vi "SVFA Zoom Cross Spectrum (Real-Im).vi"(0 "scaled signal X [EUx]":waveform(dbl)={"t0"=timestamp(0 s since 1904-01-01), "dt"=1e-05, "Y"=[]}, 1 "scaled signal Y [EUy]":waveform(dbl)={"t0"=timestamp(0 s since 1904-01-01), "dt"=1e-05, "Y"=[]}, 3 "zoom settings":T7={"frequency range"={"start frequency"=1000.0, "stop frequency"=2000.0}, "window"=1, "number of lines"=400, "% overlap"=0.0} {"% overlap" min=0.0 format="%.2f"; "number of lines" min=2; "window" items=["None ", "Hanning", "Hamming", "Blackman-Harris", "Exact Blackman", "Blackman", "Flat Top", "4 Term B-Harris ", "7 Term B-Harris", "Low Sidelobe"]; "frequency range"."stop frequency" min=0.0 format="%.2f"; "frequency range"."start frequency" min=0.0 format="%.2f"}, 5 "error in (no error)":errorcluster, 7 "averaging parameters":T9={"averaging mode"=enum."No averaging", "weighting mode"=enum."Exponential", "number of averages"=10, "linear mode"=enum."One shot"} {"number of averages" min=1 step=1}, 9 "restart averaging (F)":bool) -> (11 "averaging done":bool, 12 "new spectrum available":bool, 13 "averages completed":dbl, 14 "real part [EUx EUy rms]":cluster{"f0":dbl, "df":dbl, "real part":dbl[]} {"real part" format="%.2p"; "df" format="%.2p"; "f0" format="%.2p"}, 16 "imaginary part [EUx EUy rms]":T8 {"imaginary part" format="%.2p"; "df" format="%.2p"; "f0" format="%.2p"}, 17 "unit label":string, 18 "spectrum info":T1={"channel name"="", "description"="", "x-axis units"=1, "spectral info"={"spectrum type"=enum."Power [Magnitude^2]", "linear/dB"=enum."linear", "window"=0, "window size"=0, "FFT size"=0}, "engineering units"=0, "custom label"="", "dB reference [EU]"=0.0, "peak units"=enum."rms", "weighting filter"=0, "spectral density?"=FALSE, "unit label"="", "spectrum skewed?"=FALSE, "complimentary spectrum units"=enum."none"} {"x-axis units" items=["Time (s)"=0, "Frequency-CB (Hz)"=1, "Frequency-CPB (Hz)"=1248, "Frequency-Arbitrary (Hz)"=2357, "Quefrency (s)"=2, "Revolutions (rev)"=3, "Order"=4, "Speed (RPM)"=11, "Speed (rad/s)"=21, "Index"=65535]; "weighting filter" items=["Linear", "A-weighting", "B-weighting", "C-weighting", "ITU-R 468-4", "Dolby", "CCITT", "C-message", "Wb", "Wc", "Wd", "We", "Wf", "Wh", "Wj", "Wk", "Wm", "AES17 20 kHz lowpass", "AES17 40 kHz lowpass", "AES17 20 kHz highpass", "AES17 40 kHz highpass"]; "dB reference [EU]" format="%.2f"; "engineering units" items=["custom..."=0, "V"=1, "A"=21, "C"=30, "pC"=31, "s"=32, "-"=29, "Pa"=2, "N"=20, "g"=3, "m/s^2"=4, "m/s"=5, "m"=6, "mm/s"=12, "mm"=13, "micron/s"=14, "micron"=15, "in/s^2"=7, "in/s"=8, "in"=9, "mil/s"=10, "mil"=11, "rad/s^2"=16, "rad/s"=17, "rad"=18, "deg/s^2"=26, "deg/s"=27, "deg"=28, "RPM"=22, "cycle/s^2"=23, "Hz"=24, "cycle"=25, "strain"=19]; "spectral info"."window" items=["None "=0, "Hanning"=1, "Hamming"=2, "Blackman-Harris"=3, "Exact Blackman"=4, "Blackman"=5, "Flat Top"=6, "4 Term B-Harris "=7, "7 Term B-Harris"=8, "Low Sidelobe"=9, "Force - Exponential"=10, "Gaussian"=62]}, 19 "error out":errorcluster)   [LabVIEW 2017]
doc: "Computes the zoom cross power spectrum of <B>scaled signal X [EUx]</B>, <B>scaled signal Y [EUy]</B>, and <B>zoom settings</B>. Results are returned as real part and imaginary part. Data accumulates each time the VI is called. However, it returns a new spectrum only when sufficient data accumulates. Indicators and subsequent processing should only be called when <B>new spectrum available</B> is TRUE."
uses:
  <vilib>/addons/_NISVFA/_Shared subVIs/Controls/svc_Spectrum Info.ctl
  <vilib>/addons/_NISVFA/_Shared subVIs/Controls/svc_X-Axis Units.ctl
  <vilib>/addons/_NISVFA/_Shared subVIs/Controls/svc_Spectrum Type.ctl
  <vilib>/addons/_NISVFA/_Shared subVIs/Controls/svc_Engineering Units Text Ring.ctl
  <vilib>/addons/_NISVFA/_Shared subVIs/Controls/svc_Weighting Filter Text Ring.ctl
  <vilib>/addons/_NISVFA/_Shared subVIs/Controls/svc_Complimentary Spectrum Units.ctl
  <vilib>/addons/_NISVFA/_Shared subVIs/Spectrum Averaging/svfa_Reset Averaging State Info.vi
  <vilib>/addons/_NISVFA/_Shared subVIs/Spectrum Averaging/svfa_Average Array with Avg Checks (complex) No State.vi
  <vilib>/addons/_NISVFA/_Shared subVIs/Spectrum Averaging/svfa_Average Array (complex) No State.vi
  <vilib>/addons/_NISVFA/_Shared subVIs/Spectrum Averaging/svfa_No Average Array (complex).vi
  <vilib>/addons/_NISVFA/_Shared subVIs/Spectrum Averaging/svfa_Average Array (complex).vi
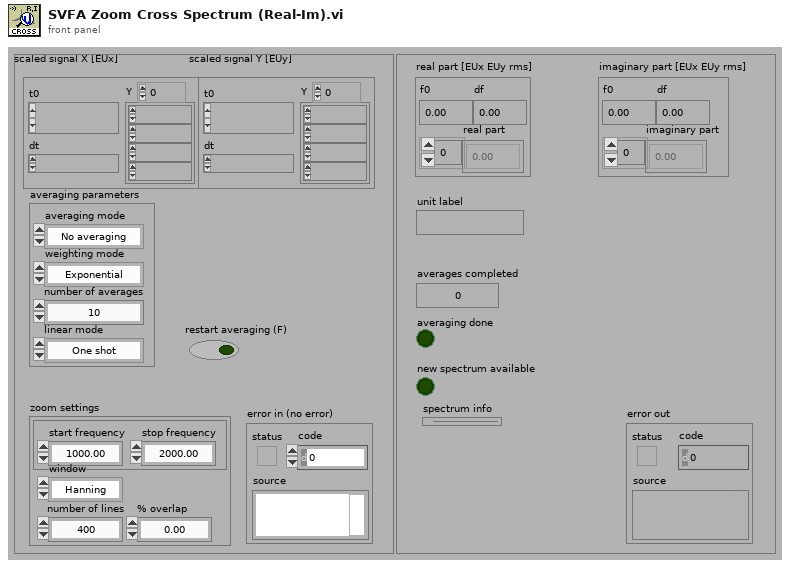
[diagram p1: front panel]
types:
  T1 = typedef "svc_Spectrum Info.ctl" = cluster{"channel name":string, "description":string, "x-axis units":T2, "spectral info":cluster{"spectrum type":T3, "linear/dB":enum16{"linear", "dB"}, "window":u16, "window size":i32, "FFT size":i32}, "engineering units":T4, "custom label":string, "dB reference [EU]":dbl, "peak units":enum16{"rms", "peak", "peak-peak"}, "weighting filter":T5, "spectral density?":bool, "unit label":string, "spectrum skewed?":bool, "complimentary spectrum units":T6}
  T2 = typedef "svc_X-Axis Units.ctl" = u16
  T3 = typedef "svc_Spectrum Type.ctl" = enum16{"FFT Spectrum [complex]", "Amplitude [Magnitude]", "Power [Magnitude^2]", "Cross Spectrum [complex]", "Frequency Response [Complex]"}
  T4 = typedef "svc_Engineering Units Text Ring.ctl" = u16
  T5 = typedef "svc_Weighting Filter Text Ring.ctl" = u16
  T6 = typedef "svc_Complimentary Spectrum Units.ctl" = enum16{"none", "radians", "degrees", "cycles", "imaginary"}
  T7 = cluster{"frequency range":cluster{"start frequency":dbl, "stop frequency":dbl}, "window":u16, "number of lines":i32, "% overlap":dbl}
  T8 = cluster{"f0":dbl, "df":dbl, "imaginary part":dbl[]}
  T9 = cluster{"averaging mode":enum16{"No averaging", "Vector averaging", "RMS averaging", "Peak hold"}, "weighting mode":enum16{"Linear", "Exponential"}, "number of averages":u32, "linear mode":enum16{"One shot", "Auto restart"}}
  T10 = enum16{"Restart processing", "Continue processing", "Skip processing"}
  T11 = enum16{"Cross spectrum", "Frequency response", "Coherent output power"}
  T12 = enum16{"No averaging", "Vector averaging", "RMS averaging", "Peak hold"}
  T13 = cluster{"zoom settings":cluster{"center frequency":dbl, "zoom":i32, "trim":dbl}, "FFT settings":cluster{"window":enum16{"None ", "Hanning", "Hamming", "Blackman-Harris", "Exact Blackman", "Blackman", "Flat Top", "4 Term B-Harris ", "7 Term B-Harris", "Low Sidelobe"}, "window size":i32, "FFT size":i32, "%overlap":dbl}}
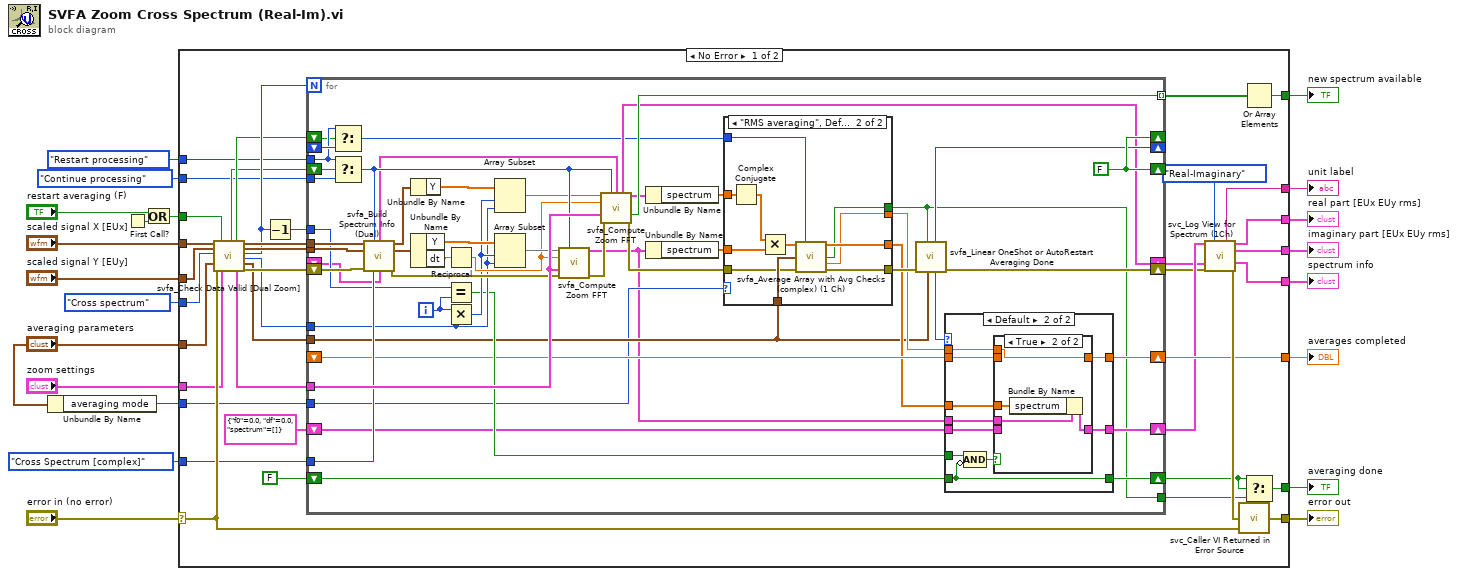
[diagram p0: block diagram]
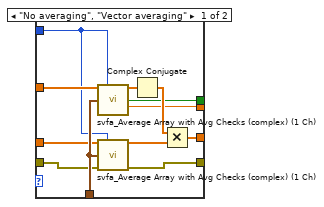
[diagram p2: hidden frame]
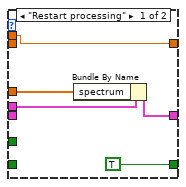
[diagram p3: hidden frame]
diagram:
  n1 = Unbundle By Name("averaging parameters") -> ("averaging mode"=w15:T12)
  n2 = First Call?() -> (First Call?: T/F=w21:bool)
  n3 = Or(x="restart averaging (F)", y=w21) -> (x .or. y?=w14:bool)
  n4 = case shown="No Error" "error in (no error)" {
    selector: "error in (no error)" -> [w50 w156]
    tunnel: "scaled signal X [EUx]" -> [w60 _]
    tunnel: "scaled signal Y [EUy]" -> [w59 _]
    tunnel: [w56 _] -> w5
    tunnel: [w55 _] -> w4
    tunnel: [w51 w156] -> w2
    tunnel: [w23 _] -> w7
    tunnel: w14 -> [w57 _]
    tunnel: "zoom settings" -> [w48 _]
    tunnel: [w25 _] -> w9
    tunnel: [w45 _] -> w8
    tunnel: [w54 _] -> w3
    tunnel: [w53 _] -> w6
    tunnel: "averaging parameters" -> [w58 _]
    tunnel: T11."Cross spectrum" ("measurement") -> [w47 _]
    tunnel: svc_Spectrum_Type."Cross Spectrum [complex]" ("spectrum type") -> [w34 _]
    tunnel: w15 -> [w33 _]
    tunnel: T10."Restart processing" ("processing control") -> [w30 _]
    tunnel: T10."Continue processing" ("processing control") -> [w29 _]
    frame No Error {
      n5 = call <vilib>:"svfa_Check Data Valid [Dual Zoom].vi"("stimulus [X]"=w60, "response [Y]"=w59, "measurement"=w47, "averaging parameters"=w58, "error in (no error)"=w50, "restart averaging (F)"=w57, "zoom settings"=w48) -> ("reset processing"=w31:bool, "restart averaging"=w32:bool, "zoom FFT settings"=w35:T13, "dup stimulus [X]"=w41:waveform(dbl), "dup response [Y]"=w40:waveform(dbl), "iterations"=w37:i32, "maximum block size"=w28:i32, "dup averaging parameters"=w38:T9, "error out"=w39:errorcluster)  [unwired: 3 in, 1 out]
      n6 = Decrement(x=w37) -> (x-1=w36:i32)
      n7 = for {
        N: w37 -> [_]
        shift-left: cluster{"f0":dbl, "df":dbl, "spectrum":cdb[]} {"f0"=0.0, "df"=0.0, "spectrum"=[]} ("FFT spectrum") -> [w77]
        shift-right: [w78] -> w44
        tunnel: w38 -> [w66]
        tunnel: [w68] -> w22
        tunnel: [w76] -> w46 mode=indexing
        tunnel: w40 -> [w106]
        tunnel: w41 -> [w107]
        shift-right: [w74] -> w43
        shift-left: _ -> [w73]
        shift-right: [w84] -> _
        shift-left: _ -> [w98]
        tunnel: w36 -> [w92]
        tunnel: w35 -> [w110]
        tunnel: w34 -> [w101]
        tunnel: w33 -> [w65]
        shift-right: [w111] -> w42
        shift-left: w39 -> [w102]
        shift-right: [w80] -> w45
        shift-left: _ -> [w79]
        shift-right: [w94] -> _
        shift-left: w32 -> [w96]
        shift-right: [w94] -> _
        shift-left: w31 -> [w100]
        tunnel: w30 -> [w97]
        tunnel: w29 -> [w99]
        tunnel: w28 -> [w85]
        shift-right: [w82] -> w24
        shift-left: FALSE ("restart averaging") -> [w81]
        i -> [w93]
        w94 = FALSE ("reset processing")
        n8 = Select(t=w97, s=w96, f=w98) -> (s? t:f=w72:T10)
        n9 = Select(t=w97, s=w100, f=w99) -> (s? t:f=w95:T10)
        n10 = call <vilib>:"svfa_Build Spectrum Info (Dual).vi"("scaled signal  X [EU]"=w107, "processing control"=w95, "scaled signal  Y [EU]"=w106, "error in (no error)"=w102, "spectrum type"=w101, "spectrum info in"=w73) -> ("spectrum info out"=w75:T1, "dup scaled signal  X [EU]"=w105:waveform(dbl), "dup scaled signal  Y [EU]"=w104:waveform(dbl), "error out"=w103:errorcluster)  [unwired: 5 in, 1 out]
        n11 = Unbundle By Name ("Get Waveform Components")(w105) -> ("Y"=w91:dbl[])
        n12 = Unbundle By Name ("Get Waveform Components")(w104) -> ("Y"=w89:dbl[], "dt"=w109:dbl)
        n13 = Reciprocal(x=w109) -> (1/x=w87:dbl)
        n14 = Equal?(x=w92, y=w93) -> (x = y?=w83:bool)
        n15 = Multiply(x=w93, y=w85) -> (x*y=w86:i32)
        n16 = Array Subset(array=w91, index=w86, length=w85) -> (w90:dbl[])
        n17 = Array Subset(array=w89, index=w86, length=w85) -> (w88:dbl[])
        n18 = call <vilib>:"svfa_Compute Zoom FFT.vi"("x"=w88, "processing control"=w95, "fs"=w87, "zoom FFT settings"=w110, "error in (no error)"=w103) -> ("FFT spectrum"=w64:cluster{"f0":dbl, "df":dbl, "spectrum":cdb[]}, "error out"=w108:errorcluster)  [unwired: 6 in, 3 out]
        n19 = call <vilib>:"svfa_Compute Zoom FFT.vi"("x"=w90, "processing control"=w95, "spectrum info"=w75, "fs"=w87, "zoom FFT settings"=w110, "error in (no error)"=w108) -> ("spectrum info out"=w74:T1, "FFT spectrum"=w62:cluster{"f0":dbl, "df":dbl, "spectrum":cdb[]}, "spectrum ready"=w76:bool, "error out"=w71:errorcluster)  [unwired: 5 in, 1 out]
        n20 = Unbundle By Name(w62) -> ("spectrum"=w61:cdb[])
        n21 = Unbundle By Name(w64) -> ("spectrum"=w63:cdb[])
        n22 = case shown="\"RMS averaging\", Default" w65 {
          tunnel: [w114 w130] -> w67
          tunnel: [w115 w131] -> w68
          tunnel: w66 -> [w118 w128]
          tunnel: w61 -> [w117 w125]
          tunnel: w63 -> [w116 w124]
          tunnel: [w122 w132] -> w69
          tunnel: w71 -> [w113 w127]
          tunnel: [w119 w126] -> w70
          tunnel: w72 -> [w112 w129]
          frame "No averaging", "Vector averaging" {
            n23 = call <vilib>:"svfa_Average Array with Avg Checks (complex) (1 Ch).vi"("spectrum"=w117, "processing control"=w112, "averaging parameters"=w118) -> ("average spectrum"=w121:cdb[], "averaging done"=w115:bool, "averages completed"=w114:dbl)  [unwired: 8 in, 2 out]
            n24 = call <vilib>:"svfa_Average Array with Avg Checks (complex) (1 Ch).vi"("spectrum"=w116, "processing control"=w112, "averaging parameters"=w118, "error in (no error)"=w113) -> ("average spectrum"=w120:cdb[], "error out"=w119:errorcluster)  [unwired: 7 in, 3 out]
            n25 = Complex Conjugate(1:w121) -> (0:w123:cdb[])
            n26 = Multiply(x=w123, y=w120) -> (x*y=w122:cdb[])
          }
          frame "RMS averaging", Default {
            n27 = Complex Conjugate(1:w125) -> (0:w134:cdb[])
            n28 = Multiply(x=w134, y=w124) -> (x*y=w133:cdb[])
            n29 = call <vilib>:"svfa_Average Array with Avg Checks (complex) (1 Ch).vi"("spectrum"=w133, "processing control"=w129, "averaging parameters"=w128, "error in (no error)"=w127) -> ("average spectrum"=w132:cdb[], "averaging done"=w131:bool, "averages completed"=w130:dbl, "error out"=w126:errorcluster)  [unwired: 7 in, 1 out]
          }
        }
        n30 = call <vilib>:"svfa_Linear OneShot or AutoRestart Averaging Done.vi"("averaging parameters"=w66, "averaging done"=w68, "error in (no error)"=w70) -> ("error out"=w111:errorcluster, "processing control"=w84:T10)  [unwired: 7 in]
        n31 = case shown="Default" w84 {
          tunnel: [TRUE ("restart averaging") w147] -> w82
          tunnel: w81 -> [_ w147]
          tunnel: w83 -> [_ w149]
          tunnel: [w138 w146] -> w80
          tunnel: w79 -> [_ w145]
          tunnel: w67 -> [w138 w144]
          tunnel: w64 -> [w135 w140]
          tunnel: w69 -> [w137 w142]
          tunnel: [w136 w143] -> w78
          tunnel: w77 -> [_ w141]
          frame "Restart processing" {
            n32 = Bundle By Name(cluster=w135, "spectrum"=w137) -> (w136:cluster{"f0":dbl, "df":dbl, "spectrum":cdb[]})
          }
          frame Default {
            n33 = Compound Arithmetic op=AND(w149, invert w147) -> (w148:bool)
            n34 = case shown="True" w148 {
              tunnel: [w151 w155] -> w146
              tunnel: w145 -> [w151 _]
              tunnel: w144 -> [_ w155]
              tunnel: w140 -> [_ w152]
              tunnel: [w150 w154] -> w143
              tunnel: w142 -> [_ w153]
              tunnel: w141 -> [w150 _]
              frame False {
              }
              frame True {
                n35 = Bundle By Name(cluster=w152, "spectrum"=w153) -> (w154:cluster{"f0":dbl, "df":dbl, "spectrum":cdb[]})
              }
            }
          }
        }
      }
      n36 = call <vilib>:"svc_Log View for Spectrum (1Ch).vi"("complex spectrum"=w44, "View"=enum16{"Mag-Phase", "Real-Imaginary"}."Real-Imaginary", "spectrum info in"=w43, "error in (no error)"=w42) -> ("unit label [mag or real]"=w53:string, "magnitude or real"=w56:cluster{"f0":dbl, "df":dbl, dbl[]}, "phase or imag"=w55:cluster{"f0":dbl, "df":dbl, dbl[]}, "spectrum info out"=w54:T1, "error out"=w52:errorcluster)  [unwired: 6 in, 1 out]
      n37 = call <vilib>:"svc_Caller VI Returned in Error Source.vi"("warning input to caller"=w50, "error in (no error)"=w52) -> ("error out"=w51:errorcluster)  [unwired: 3 in]
      n38 = Or Array Elements(Boolean array=w46) -> (logical OR=w25:bool)
      n39 = Select(t=w24, s=w24, f=w22) -> (s? t:f=w23:bool)
    }
    frame Error {
    }
  }
  "error out" <- w2
  "imaginary part [EUx EUy rms]" <- w4
  "real part [EUx EUy rms]" <- w5
  "unit label" <- w6
  "averages completed" <- w8
  "averaging done" <- w7
  "new spectrum available" <- w9
  "spectrum info" <- w3
